vi "RecipeDataReadingStringToClusterFormar.vi"(11 "StringFormat":string[](array[string])) -> (3 "ClusterFormat":T1)   [LabVIEW 2014]
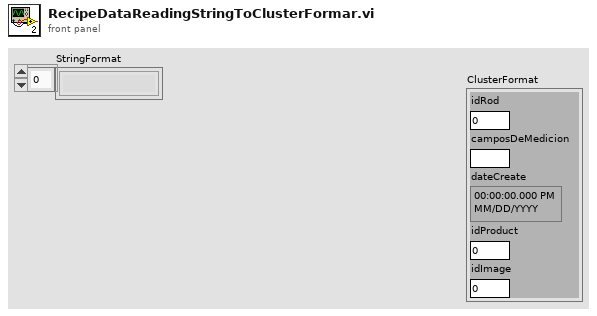
[diagram p1: front panel]
types:
  T1 = cluster{"idRod":dbl, "camposDeMedicion":string, "dateCreate":timestamp, "idProduct":dbl, "idImage":dbl}
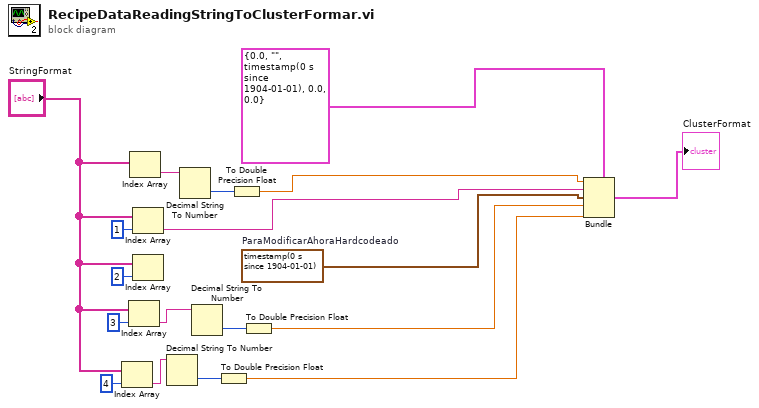
[diagram p0: block diagram]
diagram:
  w7 = timestamp(0 s since 1904-01-01)  # ParaModificarAhoraHardcodeado
  n1 = Index Array(array="StringFormat", index=4) -> (element=w2:string)
  n2 = Index Array(array="StringFormat", index=3) -> (element=w5:string)
  n3 = Index Array(array="StringFormat") -> (element=w18:string)  [unwired: 1 in]
  n4 = Index Array(array="StringFormat", index=1) -> (element=w13:string)
  n5 = Index Array(array="StringFormat", index=2) -> ()  [unwired: 1 out]
  n6 = Decimal String To Number(string=w2) -> (number=w3:i32)  [unwired: 2 in, 1 out]
  n7 = Decimal String To Number(string=w18) -> (number=w15:i32)  [unwired: 2 in, 1 out]
  n8 = Decimal String To Number(string=w5) -> (number=w6:i32)  [unwired: 2 in, 1 out]
  n9 = To Double Precision Float(number=w3) -> (double precision float=w1:dbl)
  n10 = To Double Precision Float(number=w15) -> (double precision float=w14:dbl)
  n11 = To Double Precision Float(number=w6) -> (double precision float=w4:dbl)
  n12 = Bundle(cluster=T1 {"idRod"=0.0, "camposDeMedicion"="", "dateCreate"=timestamp(0 s since 1904-01-01), "idProduct"=0.0, "idImage"=0.0} ("ClusterFormat 2"), "idRod"=w14, "camposDeMedicion"=w13, "dateCreate"=w7, "idProduct"=w4, "idImage"=w1) -> (→"ClusterFormat":T1)
